vi "Get Other E2E Nodes Details.vi"(8 "error in (no error)":errorcluster, 10 "Other E2E editor nodes":refnum<data-value>[](array[refnum]), 11 "E2E editor node in":refnum<data-value>) -> (0 "error out":errorcluster, 2 "E2E Nodes by Line":T1[](array[typedef]), 3 "E2E editor node out":refnum<data-value>)   [LabVIEW 2015, in "E2E Tag Exchange editor node.lvclass"]
uses:
  E2E Tag Exchange editor node.lvclass
  Pairing Details Line.ctl
  module/configuration/Runtime Implementation.ctl
  <vilib>/NI/Configuration Framework/Node/NISE_CEF_Node.lvclass
  module/configuration/E2E Tag Exchange configuration.lvclass
  module/configuration/E2E Tag Exchange configuration.lvclass/E2E Tag Exchange configuration.ctl
  <vilib>/NI/Configuration Framework/serializable configuration/NISE_CEF_serializable configuration.lvclass/NISE_CEF_serializable configuration.ctl
  <vilib>/NI/DCAF/Tag Editor Core/Configuration Editor/Classes/Module editor node/Read display name.vi
  <vilib>/Utility/LVClass/Get LV Class Name.vi
  <vilib>/NI/Configuration Framework/error generator/NISE_error generator.vi
  <vilib>/NI/Configuration Framework/serializable configuration/NISE_CEF_serializable configuration.lvclass
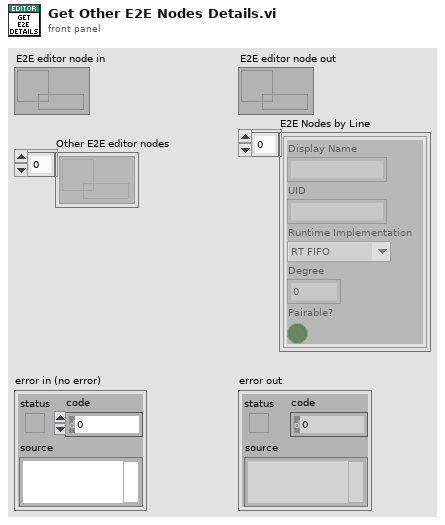
[diagram p1: front panel]
types:
  T1 = typedef "E2E Tag Exchange editor node.lvclass/Pairing Details Line.ctl" = cluster{"Display Name":string, "UID":string, "Runtime Implementation":T2, "Degree":i32, "Pairable?":bool}
  T2 = typedef "E2E Tag Exchange configuration.lvclass/Runtime Implementation.ctl" = enum16{"RT FIFO", "UDP"}
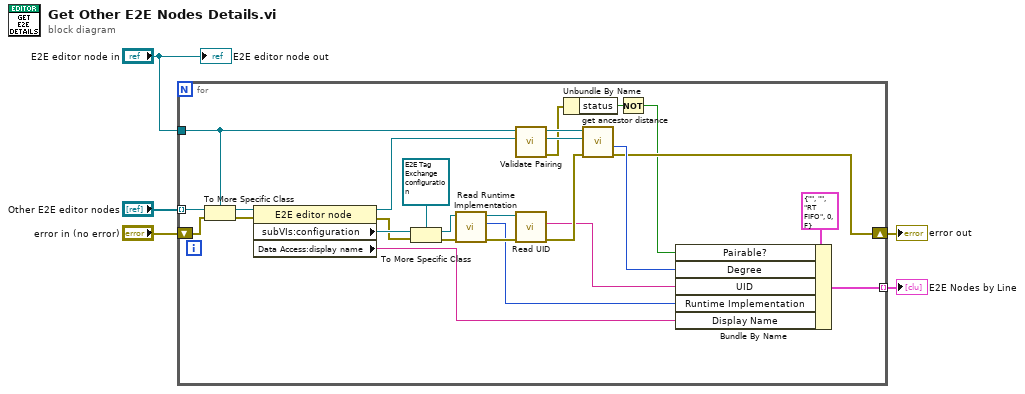
[diagram p0: block diagram]
diagram:
  n1 = for {
    tunnel: "Other E2E editor nodes" -> [w31] mode=indexing
    shift-right: [w9] -> w5
    shift-left: "error in (no error)" -> [w29]
    tunnel: "E2E editor node in" -> [w13]
    tunnel: [w17] -> w4 mode=indexing
    n2 = To More Specific Class(target class=w13, reference=w31, error in=w29) -> (specific class reference=w30:refnum<data-value>, error out=w28:errorcluster)
    n3 = property class="E2E editor node"(reference=w30, error in=w28) -> (reference out=w12:refnum<data-value>, error out=w25:errorcluster, "subVIs:configuration"=w27:refnum<class "NISE_CEF_serializable configuration.lvclass">, "Data Access:display name"=w14:string)
    n4 = To More Specific Class(target class=refnum<class "E2E Tag Exchange configuration.lvclass"> refnum ("E2E Tag Exchange configuration in"), reference=w27, error in=w25) -> (specific class reference=w23:refnum<class "E2E Tag Exchange configuration.lvclass">, error out=w24:errorcluster)
    n5 = call "Read Runtime Implementation.vi"("error in (no error)"=w24, "E2E Tag Exchange configuration in"=w23) -> ("error out"=w21:errorcluster, "Runtime Implementation"=w15:T2, "E2E Tag Exchange configuration out"=w22:refnum<class "E2E Tag Exchange configuration.lvclass">)  [unwired: 7 in]
    n6 = call "Validate Pairing.vi"("E2E node 2"=w12, "E2E node 1"=w13) -> ("error out"=w8:errorcluster, "E2E node 2 out"=w10:refnum<data-value>, "E2E node 1 out"=w11:refnum<data-value>)  [unwired: 7 in]
    n7 = call <vilib>:"Read UID.vi"("error in"=w21, "configuration in"=w22) -> ("error out"=w20:errorcluster, "instance id"=w19:string)  [unwired: 7 in, 1 out]
    n8 = Unbundle By Name(w8) -> ("status"=w7:bool)
    n9 = call "get ancestor distance.vi"("error in (no error)"=w20, "node 2"=w10, "node 1"=w11) -> ("error out"=w9:errorcluster, "Degree out"=w16:i32)  [unwired: 5 in, 2 out]
    n10 = Not(x=w7) -> (.not. x?=w6:bool)
    n11 = Bundle By Name(cluster=T1 {"Display Name"="", "UID"="", "Runtime Implementation"=enum."RT FIFO", "Degree"=0, "Pairable?"=FALSE}, "Pairable?"=w6, "Degree"=w16, "UID"=w19, "Runtime Implementation"=w15, "Display Name"=w14) -> (w17:T1)
  }
  "error out" <- w5
  "E2E Nodes by Line" <- w4
  "E2E editor node out" <- "E2E editor node in"
